vi "Read Magnet Field.vi"(8 "error in (no error)":errorcluster, 11 "instrument.PPMS2 in":refnum<class "instrument.PPMS2.lvclass">) -> (0 "error out":errorcluster, 1 "Ramping?":bool, 2 "Field (T)":dbl, 3 "instrument.PPMS2 out":refnum<class "instrument.PPMS2.lvclass">)   [LabVIEW 2016, in "instrument.PPMS2.lvclass"]
uses:
  instrument.PPMS2.lvclass
  levylab_inst/Instrument/Instrument.lvclass
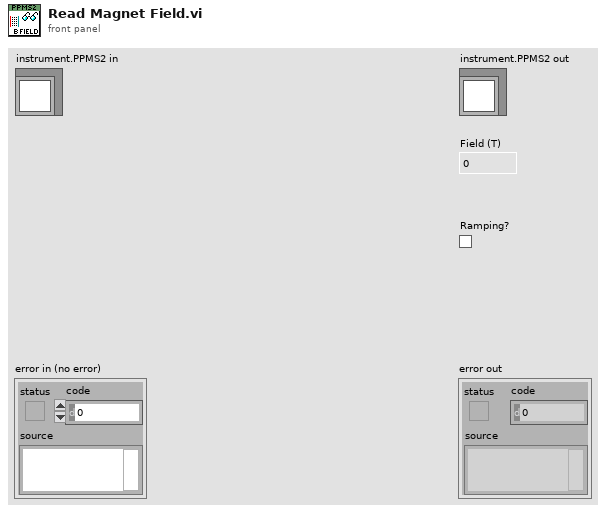
[diagram p1: front panel]
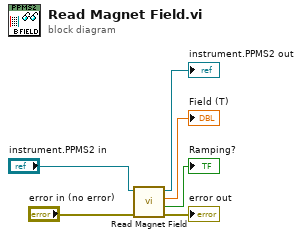
[diagram p0: block diagram]
diagram:
  n1 = call-parent "Read Magnet Field.vi"("error in (no error)"="error in (no error)", "Instrument in"="instrument.PPMS2 in") -> ("error out"=→"error out":errorcluster, "Ramping?"=→"Ramping?":bool, "Field (T)"=→"Field (T)":dbl, "Instrument out"=→"instrument.PPMS2 out":refnum<class "instrument.PPMS2.lvclass">)  [unwired: 6 in]
